vi "LabelCtl.vi"(8 "error in":errorcluster caption="错误输入", 10 "测试参数":T2={"帧ID1"=0, "等待延时"=0, "间隔延时"=0, "总时间"=0, "总次数"=0, "发送数据1"="", "接收数据1"="", "发送数据2"="", "接收数据2"="", "CAN盒类型"=3, "帧ID2"=0, "同步启动个数"=8, "模式"=enum."整体", "Baud"=12} {"Baud" items=["250k bps"=10, "10k bps"=2, "5k bps"=1, "50k bps"=5, "40k bps"=4, "20k bps"=3, "80k bps"=6, "100k bps"=7, "125k bps"=8, "200k bps"=9, "400k bps"=11, "500k bps"=12, "666k bps"=13, "800k bps"=14, "1000k bps"=15]; "帧ID2" format="%.0x"; "CAN盒类型" items=["PCI-CAN200"=7, "USB-CAN"=2, "USB-CAN200"=3]; "帧ID1" format="%.0x"}, 11 "LabelIn":T3) -> (0 "error out":errorcluster caption="错误输出", 2 "Value":string[](array[string]), 3 "LabelText":string[](array[string]))   [LabVIEW 2013]
uses:
  USBCAN/DevType.ctl
panel:
  # "ms"
  # "ms"
  # "s"
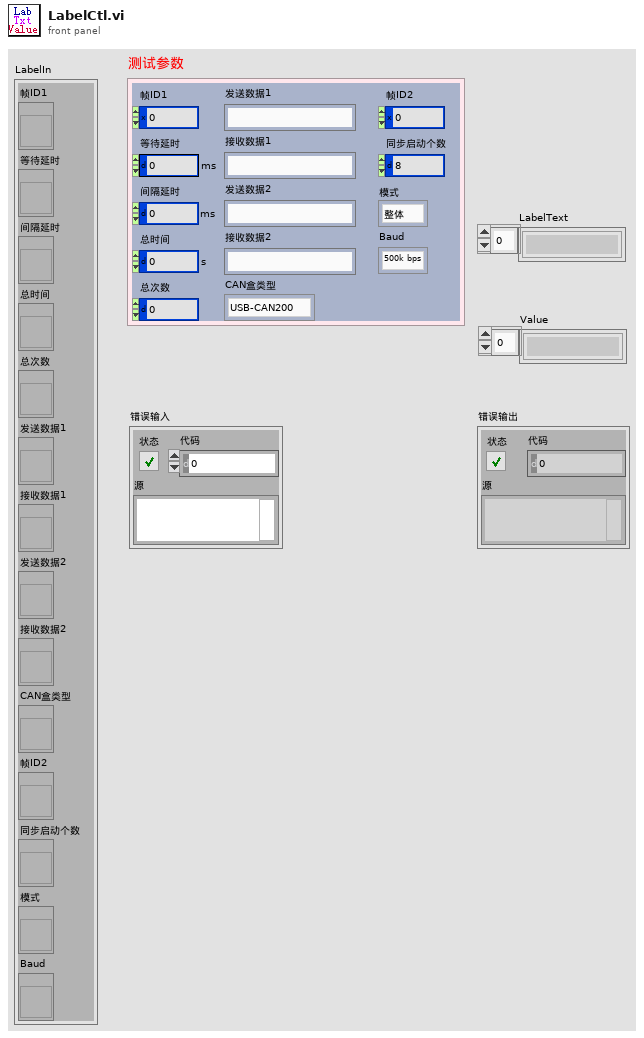
[diagram p1: front panel]
types:
  T1 = typedef "DevType.ctl" = u16
  T2 = cluster{"帧ID1":u32, "等待延时":u32, "间隔延时":u32, "总时间":u32, "总次数":u32, "发送数据1":string, "接收数据1":string, "发送数据2":string, "接收数据2":string, "CAN盒类型":T1, "帧ID2":u32, "同步启动个数":u8, "模式":enum16{"整体", "单个"}, "Baud":u8}
  T3 = cluster{"帧ID1":refnum<vi>, "等待延时":refnum<vi>, "间隔延时":refnum<vi>, "总时间":refnum<vi>, "总次数":refnum<vi>, "发送数据1":refnum<vi>, "接收数据1":refnum<vi>, "发送数据2":refnum<vi>, "接收数据2":refnum<vi>, "CAN盒类型":refnum<vi>, "帧ID2":refnum<vi>, "同步启动个数":refnum<vi>, "模式":refnum<vi>, "Baud":refnum<vi>}
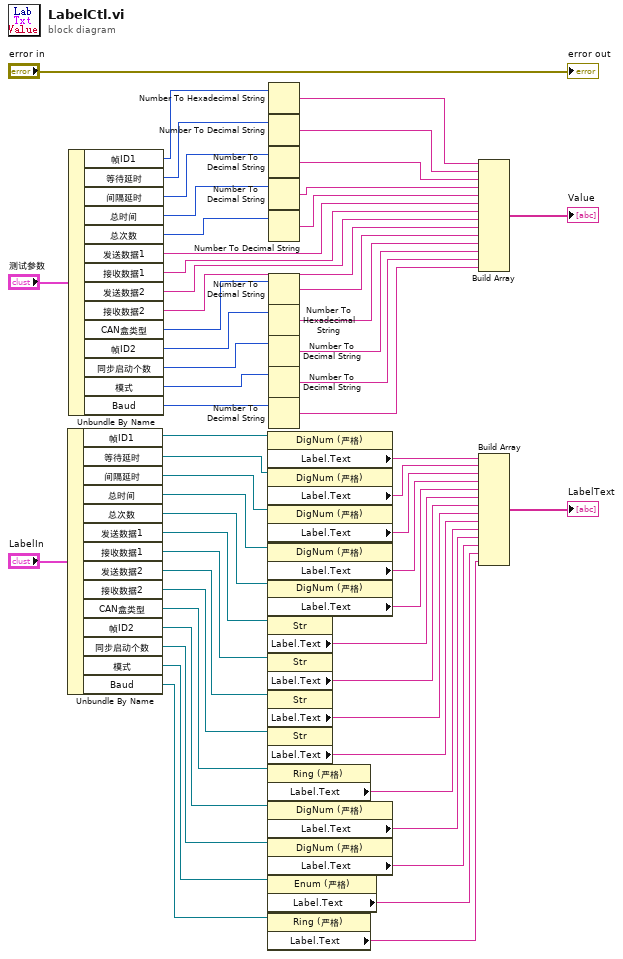
[diagram p0: block diagram]
diagram:
  n1 = Unbundle By Name("LabelIn") -> ("帧ID1"=w56:refnum<vi>, "等待延时"=w55:refnum<vi>, "间隔延时"=w54:refnum<vi>, "总时间"=w53:refnum<vi>, "总次数"=w52:refnum<vi>, "发送数据1"=w51:refnum<vi>, "接收数据1"=w50:refnum<vi>, "发送数据2"=w49:refnum<vi>, "接收数据2"=w48:refnum<vi>, "CAN盒类型"=w47:refnum<vi>, "帧ID2"=w46:refnum<vi>, "同步启动个数"=w45:refnum<vi>, "模式"=w44:refnum<vi>, "Baud"=w43:refnum<vi>)
  n2 = Unbundle By Name("测试参数") -> ("帧ID1"=w26:u32, "等待延时"=w25:u32, "间隔延时"=w24:u32, "总时间"=w23:u32, "总次数"=w22:u32, "发送数据1"=w11:string, "接收数据1"=w10:string, "发送数据2"=w9:string, "接收数据2"=w8:string, "CAN盒类型"=w21:T1, "帧ID2"=w20:u32, "同步启动个数"=w19:u8, "模式"=w18:enum16{"整体", "单个"}, "Baud"=w17:u8)
  n3 = property class="DigNum (严格)"(reference=w56) -> ("Label.Text"=w42:string)  [unwired: 1 in, 2 out]
  n4 = property class="DigNum (严格)"(reference=w55) -> ("Label.Text"=w41:string)  [unwired: 1 in, 2 out]
  n5 = property class="DigNum (严格)"(reference=w54) -> ("Label.Text"=w40:string)  [unwired: 1 in, 2 out]
  n6 = property class="DigNum (严格)"(reference=w53) -> ("Label.Text"=w39:string)  [unwired: 1 in, 2 out]
  n7 = property class="DigNum (严格)"(reference=w52) -> ("Label.Text"=w38:string)  [unwired: 1 in, 2 out]
  n8 = property class="Str"(reference=w51) -> ("Label.Text"=w37:string)  [unwired: 1 in, 2 out]
  n9 = property class="Str"(reference=w50) -> ("Label.Text"=w36:string)  [unwired: 1 in, 2 out]
  n10 = property class="Str"(reference=w49) -> ("Label.Text"=w35:string)  [unwired: 1 in, 2 out]
  n11 = property class="Str"(reference=w48) -> ("Label.Text"=w34:string)  [unwired: 1 in, 2 out]
  n12 = property class="Ring (严格)"(reference=w47) -> ("Label.Text"=w33:string)  [unwired: 1 in, 2 out]
  n13 = property class="DigNum (严格)"(reference=w46) -> ("Label.Text"=w32:string)  [unwired: 1 in, 2 out]
  n14 = property class="DigNum (严格)"(reference=w45) -> ("Label.Text"=w31:string)  [unwired: 1 in, 2 out]
  n15 = property class="Enum (严格)"(reference=w44) -> ("Label.Text"=w30:string)  [unwired: 1 in, 2 out]
  n16 = property class="Ring (严格)"(reference=w43) -> ("Label.Text"=w29:string)  [unwired: 1 in, 2 out]
  n17 = Number To Hexadecimal String(2:w26) -> (0:w16:string)  [unwired: 1 in]
  n18 = Number To Decimal String(number=w25) -> (decimal integer string=w15:string)  [unwired: 1 in]
  n19 = Number To Decimal String(number=w24) -> (decimal integer string=w14:string)  [unwired: 1 in]
  n20 = Number To Decimal String(number=w23) -> (decimal integer string=w13:string)  [unwired: 1 in]
  n21 = Number To Decimal String(number=w22) -> (decimal integer string=w12:string)  [unwired: 1 in]
  n22 = Number To Decimal String(number=w21) -> (decimal integer string=w7:string)  [unwired: 1 in]
  n23 = Number To Hexadecimal String(2:w20) -> (0:w6:string)  [unwired: 1 in]
  n24 = Number To Decimal String(number=w19) -> (decimal integer string=w5:string)  [unwired: 1 in]
  n25 = Number To Decimal String(number=w18) -> (decimal integer string=w4:string)  [unwired: 1 in]
  n26 = Number To Decimal String(number=w17) -> (decimal integer string=w3:string)  [unwired: 1 in]
  n27 = Build Array(w16, w15, w14, w13, w12, w11, w10, w9, w8, w7, w6, w5, w4, w3) -> (→"Value":string[])
  n28 = Build Array(w42, w41, w40, w39, w38, w37, w36, w35, w34, w33, w32, w31, w30, w29) -> (→"LabelText":string[])
  "error out" <- "error in"
